vi "svx_Polar_Get_Selector_Texts.vi"(8 "error in":errorcluster, 9 "Selector:ring Strings":T1, 11 "polar plot":T2) -> (0 "error out":errorcluster, 1 "Selector:ring Strings out":T1, 2 "update legend?":bool)   [LabVIEW 2017, in "SVX Polar Plot.xctl"]
uses:
  <vilib>/addons/_XControls/Polar Plot/SVX Polar Plot.xctl
  <vilib>/addons/_XControls/Polar Plot/subVIs/svx_Polar_Plot_Data.ctl
  <vilib>/addons/_XControls/Polar Plot/subVIs/svx_Polar_Attribute.ctl
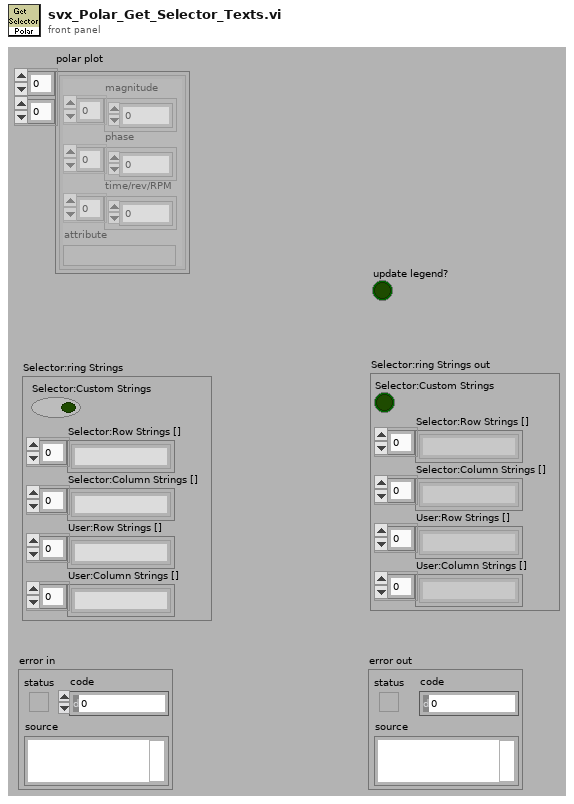
[diagram p1: front panel]
types:
  T1 = cluster{"Selector:Custom Strings":bool, "Selector:Row Strings []":string[], "Selector:Column Strings []":string[], "User:Row Strings []":string[], "User:Column Strings []":string[]}
  T2 = typedef "SVX Polar Plot.xctl/svx_Polar_Plot_Data.ctl" = cluster{"magnitude":dbl[], "phase":dbl[], "time/rev/RPM":dbl[], "attribute":variant}[][]
  T3 = typedef "SVX Polar Plot.xctl/svx_Polar_Attribute.ctl" = u16
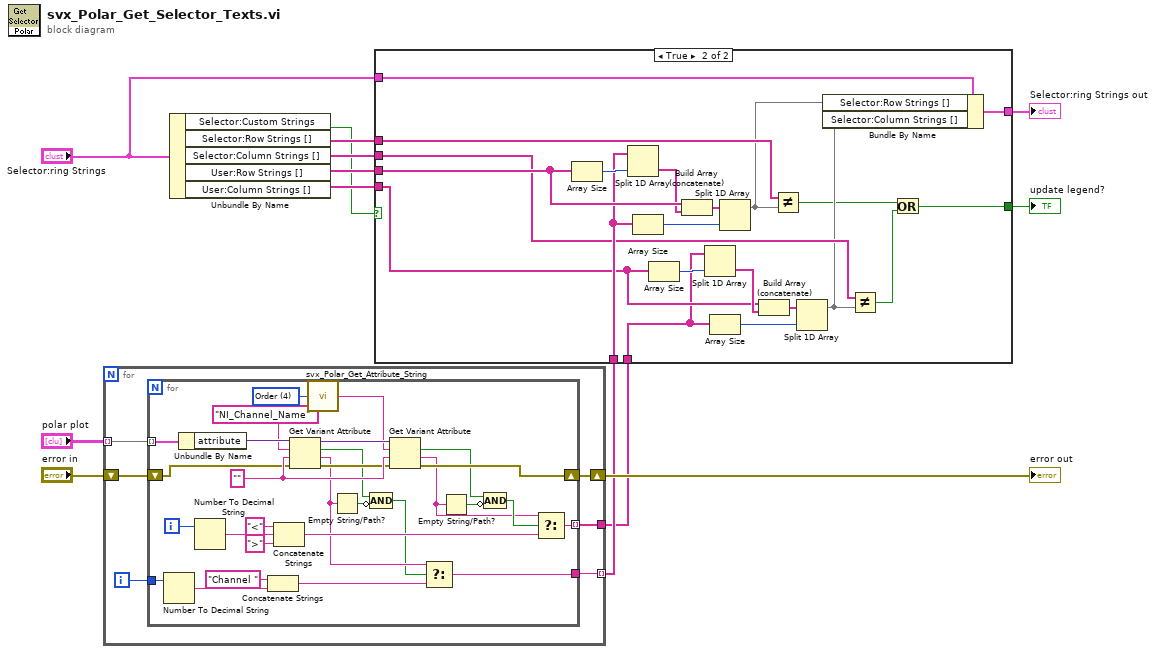
[diagram p0: block diagram]
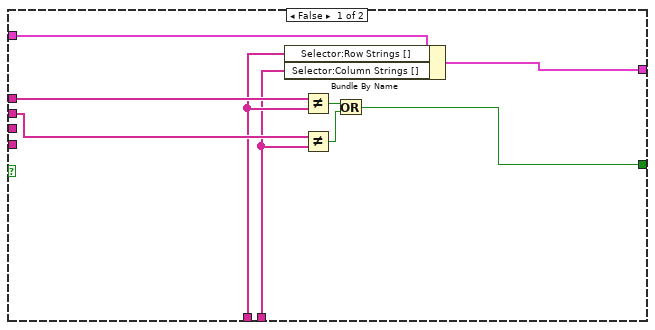
[diagram p2: hidden frame]
diagram:
  n1 = for {
    tunnel: "polar plot" -> [w19] mode=indexing
    tunnel: [w17] -> w4
    tunnel: [w16] -> w5 mode=indexing
    shift-right: [w14] -> w11
    shift-left: "error in" -> [w15]
    i -> [w18]
    n2 = for {
      tunnel: w19 -> [w48] mode=indexing
      tunnel: w18 -> [w45]
      tunnel: [w41] -> w16
      tunnel: [w33] -> w17 mode=indexing
      shift-right: [w30] -> w14
      shift-left: w15 -> [w32]
      i -> [w38]
      w21 = T3 4 items=["Pulse / Revolution", "Slope", "Threshold", "Hysteresis", "Order", "Reference Label", "Rotation Direction", "Pair String", "Polar Plot Type", "Sample Per Revolution", "Probe Angle", "Probe Angle X", "Probe Angle Y", "X Axis Unit", "OTB Plot Type"] ("SVMS attribute")
      w39 = "" ("name")
      n3 = Number To Decimal String(number=w45) -> (decimal integer string=w44:string)  [unwired: 1 in]
      n4 = Unbundle By Name(w48) -> ("attribute"=w47:variant)
      n5 = Number To Decimal String(number=w38) -> (decimal integer string=w37:string)  [unwired: 1 in]
      n6 = Concatenate Strings("Channel " ("string"), w44) -> (w42:string)
      n7 = Concatenate Strings("<" ("string"), w37, ">" ("string")) -> (w34:string)
      n8 = Get Variant Attribute(Variant=w47, name="NI_Channel_Name", default value (empty Variant)=w39, error in=w32) -> (duplicate Variant=w40:variant, found=w27:bool, value=w29:string, error out=w31:errorcluster)
      n9 = call <vilib>:"svx_Polar_Get_Attribute_String.vi"("SVMS attribute"=w21) -> ("attribute name"=w20:string)  [unwired: 4 in]
      n10 = Empty String/Path?(string/path=w29) -> (empty?=w28:bool)
      n11 = Compound Arithmetic op=AND(w27, invert w28) -> (w26:bool)
      n12 = Get Variant Attribute(Variant=w40, name=w20, default value (empty Variant)=w39, error in=w31) -> (found=w24:bool, value=w22:string, error out=w30:errorcluster)  [unwired: 1 out]
      n13 = Select(t=w29, s=w26, f=w42) -> (s? t:f=w41:string)
      n14 = Empty String/Path?(string/path=w22) -> (empty?=w23:bool)
      n15 = Compound Arithmetic op=AND(w24, invert w23) -> (w25:bool)
      n16 = Select(t=w22, s=w25, f=w34) -> (s? t:f=w33:string)
    }
  }
  "error out" <- w11
  n17 = Unbundle By Name("Selector:ring Strings") -> ("Selector:Custom Strings"=w2:bool, "Selector:Row Strings []"=w10:string[], "Selector:Column Strings []"=w9:string[], "User:Row Strings []"=w8:string[], "User:Column Strings []"=w7:string[])
  n18 = case shown="True" w2 {
    tunnel: w10 -> [w56 w72]
    tunnel: w9 -> [w55 w64]
    tunnel: w8 -> [_ w77]
    tunnel: w7 -> [_ w63]
    tunnel: "Selector:ring Strings" -> [w57 w71]
    tunnel: w5 -> [w54 w74]
    tunnel: w4 -> [w53 w62]
    tunnel: [w50 w58] -> w1
    tunnel: [w49 w69] -> w3
    frame False {
      n19 = Bundle By Name(cluster=w57, "Selector:Row Strings []"=w54, "Selector:Column Strings []"=w53) -> (w49:T1)
      n20 = Not Equal?(x=w56, y=w54) -> (x != y?=w52:bool)
      n21 = Not Equal?(x=w55, y=w53) -> (x != y?=w51:bool)
      n22 = Or(x=w52, y=w51) -> (x .or. y?=w50:bool)
    }
    frame True {
      n23 = Array Size(array=w77) -> (size(s)=w78:i32)
      n24 = Split 1D Array(array=w74, index=w78) -> (second subarray=w76:string[])  [unwired: 1 out]
      n25 = Array Size(array=w74) -> (size(s)=w73:i32)
      n26 = Array Size(array=w63) -> (size(s)=w65:i32)
      n27 = Build Array (concatenate)(w77, w76) -> (w75:string[])
      n28 = Split 1D Array(array=w62, index=w65) -> (second subarray=w66:string[])  [unwired: 1 out]
      n29 = Array Size(array=w62) -> (size(s)=w68:i32)
      n30 = Split 1D Array(array=w75, index=w73) -> (first subarray=w70:string[])  [unwired: 1 out]
      n31 = Build Array (concatenate)(w63, w66) -> (w67:string[])
      n32 = Not Equal?(x=w72, y=w70) -> (x != y?=w60:bool)
      n33 = Split 1D Array(array=w67, index=w68) -> (first subarray=w61:string[])  [unwired: 1 out]
      n34 = Bundle By Name(cluster=w71, "Selector:Row Strings []"=w70, "Selector:Column Strings []"=w61) -> (w69:T1)
      n35 = Not Equal?(x=w64, y=w61) -> (x != y?=w59:bool)
      n36 = Or(x=w60, y=w59) -> (x .or. y?=w58:bool)
    }
  }
  "update legend?" <- w1
  "Selector:ring Strings out" <- w3
